vi "Formula Node Exercise Brian Sheridan.vi"() -> ()   [LabVIEW 2014]
panel:
  out "Waveform Graph":dbl[](graph)
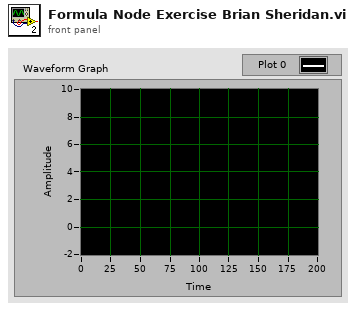
[diagram p1: front panel]
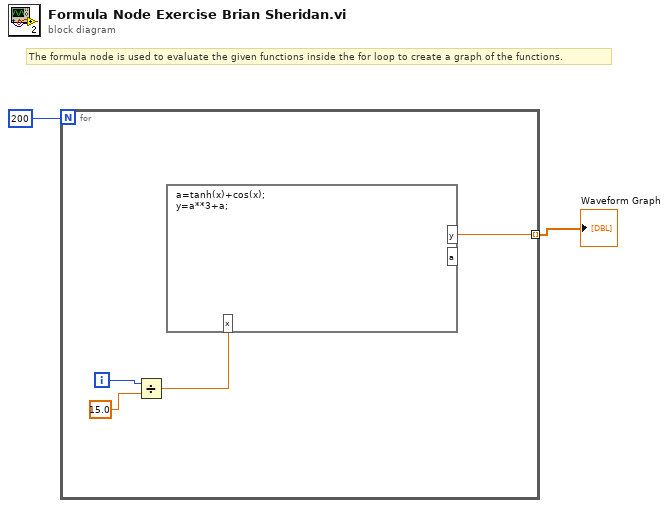
[diagram p0: block diagram]
diagram:
  # "The formula node is used to evaluate the given functions inside the for loop to create a graph of the functions."
  n1 = for {
    N: 200 -> [_]
    tunnel: [w3] -> w1 mode=indexing
    i -> [w5]
    n2 = Divide(x=w5, y=15.0) -> (x/y=w6:dbl)
    n3 = formula code="a=tanh(x)+cos(x);\ny=a**3+a;"("x"=w6) -> ("y"=w3:dbl)  [unwired: 1 out]
  }
  "Waveform Graph" <- w1
